vi "FilterCommands.vi"(8 "error in (no error)":errorcluster, 10 "CAN Frames":T1[](array[typedef]) {"payload" format="%x"; "timestamp" format="%<%.7X\n%x>T"; "type" items=["CAN Data"=0, "CAN Remote"=1, "CAN Bus Error"=2, "CAN 2.0 Data"=8, "CAN FD Data"=16, "CAN FD+BRS Data"=24, "J1939 Data"=192, "Delay"=224, "Log Trigger"=225, "Start Trigger"=226]; "identifier" format="%x"}, 11 "DAQList in":refnum<class "DAQList.lvclass">) -> (0 "error out":errorcluster, 3 "DAQList out":refnum<class "DAQList.lvclass">)   [LabVIEW 2019, in "XCP_DaqDtoId.lvlib" / "DAQList.lvclass"]
uses:
  DAQList.lvclass
  <vilib>/xnet/xnet.llb/XNET Frame CAN.ctl
  <vilib>/xnet/xnet.llb/XNET Frame Type CAN.ctl
  DAQList.lvclass/DAQList.ctl
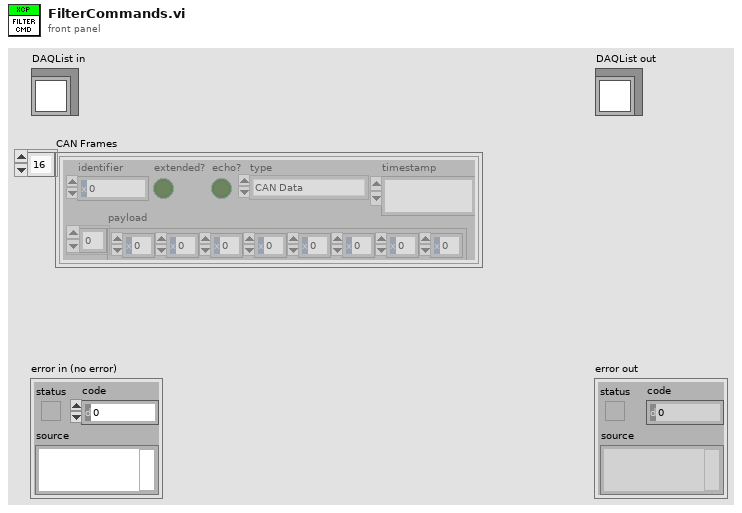
[diagram p1: front panel]
types:
  T1 = typedef "XNET Frame CAN.ctl" = cluster{"timestamp":timestamp, "payload":u8[], "identifier":u32, "type":T2, "extended?":bool, "echo?":bool}
  T2 = typedef "XNET Frame Type CAN.ctl" = u8
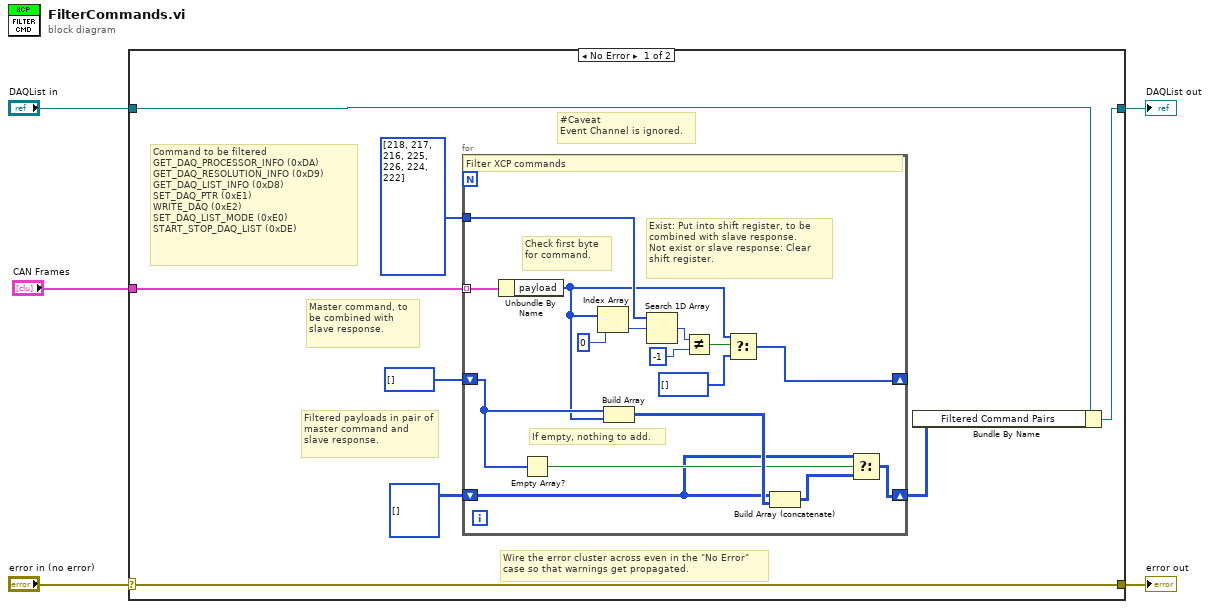
[diagram p0: block diagram]
diagram:
  n1 = case shown="No Error" "error in (no error)" {
    selector: "error in (no error)" -> [w13 w31]
    tunnel: [w13 w31] -> w4
    tunnel: [w6 w30] -> w2
    tunnel: "DAQList in" -> [w8 w30]
    tunnel: "CAN Frames" -> [w9 _]
    frame No Error {
      # "#Caveat \nEvent Channel is ignored."
      # "Filtered payloads in pair of master command and slave response."
      # "Master command, to be combined with slave response."
      # "Command to be filtered\nGET_DAQ_PROCESSOR_INFO (0xDA)\nGET_DAQ_RESOLUTION_INFO (0xD9)\nGET_DAQ_LIST_INFO (0xD8)\nSET_DAQ_PTR (0xE1)\nWRITE_DAQ (0xE2)\nSET_DAQ_LIST_MODE (0xE0)\nSTART_STOP_DAQ_LIST (0xDE)"
      # "Wire the error cluster across even in the \"No Error\"\ncase so that warnings get propagated."
      n2 = for {
        tunnel: w9 -> [w29] mode=indexing
        tunnel: u8[] [218, 217, 216, 225, 226, 224, 222] -> [w27]
        shift-right: [w22] -> _
        shift-left: u8[] [] ("payload") -> [w15]
        shift-right: [w17] -> w7
        shift-left: u8[][][] [] -> [w18]
        # "If empty, nothing to add."
        # "Exist: Put into shift register, to be combined with slave response.\nNot exist or slave response: Clear shift register."
        # "Check first byte for command."
        # "Filter XCP commands"
        n3 = Unbundle By Name(w29) -> ("payload"=w14:u8[])
        n4 = Empty Array?(array=w15) -> (empty?=w19:bool)
        n5 = Index Array(array=w14, index=0) -> (element=w26:u8)
        n6 = Build Array(w15, w14) -> (w20:u8[][])
        n7 = Search 1D Array(1D array=w27, element=w26) -> (index of element=w25:i32)  [unwired: 1 in]
        n8 = Not Equal?(x=w25, y=-1) -> (x != y?=w23:bool)
        n9 = Select(t=w14, s=w23, f=u8[] [] ("payload")) -> (s? t:f=w22:u8[])
        n10 = Build Array (concatenate)(w18, w20) -> (w16:u8[][][])
        n11 = Select(t=w18, s=w19, f=w16) -> (s? t:f=w17:u8[][][])
      }
      n12 = Bundle By Name(cluster=w8, "Filtered Command Pairs"=w7) -> (w6:refnum<class "DAQList.lvclass">)
    }
    frame Error {
    }
  }
  "error out" <- w4
  "DAQList out" <- w2
